vi "Write Library Data.vi"(4 "Library Path":path, 6 "Icon data":T1={"Text Visible?"=FALSE, "Text Opacity"=0, "Templ Visible?"=FALSE, "Templ Opacity"=0, "Relative Path from 1 to 2"=path "", "Image"=bytes[0], "All User Layers"=[], "Body Text"={"Line 1 text"="", "Line 2 text"="", "Line 3 text"="", "Line 4 text"="", "Line 1 color"=0, "Line 2 color"=0, "Line 3 color"=0, "Line 4 color"=0, "Body Text Spec"={"Font"="", "Alignment"=0, "Size"=3}, "Center text vertically"=FALSE, "Capitalize Text"=FALSE}} {"Body Text"."Body Text Spec"."Alignment" items=["left", "center", "right"]}, 8 "error in":errorcluster, 11 "Library Icon Data in":refnum<class "Library Icon Data.lvclass">) -> (0 "error out":errorcluster, 3 "Library Icon Data out":refnum<class "Library Icon Data.lvclass">)   [LabVIEW 2020, in "Library Icon Data.lvclass"]
uses:
  Library Icon Data.lvclass
  Library Icon Data.lvclass/Library Icon Data.ctl
  resource/plugins/lv_icon.lvlib
  vi.lib/LabVIEW Icon API/lv_icon/Controls/Font.ctl
  vi.lib/LabVIEW Icon API/lv_icon/Controls/Alignment.ctl
  vi.lib/LabVIEW Icon API/lv_icon/Controls/BodyText.ctl
  vi.lib/LabVIEW Icon API/lv_icon/Classes/Layer/Layer.lvclass
  vi.lib/LabVIEW Icon API/lv_icon/Controls/LabVIEW Icon Stored Information.ctl
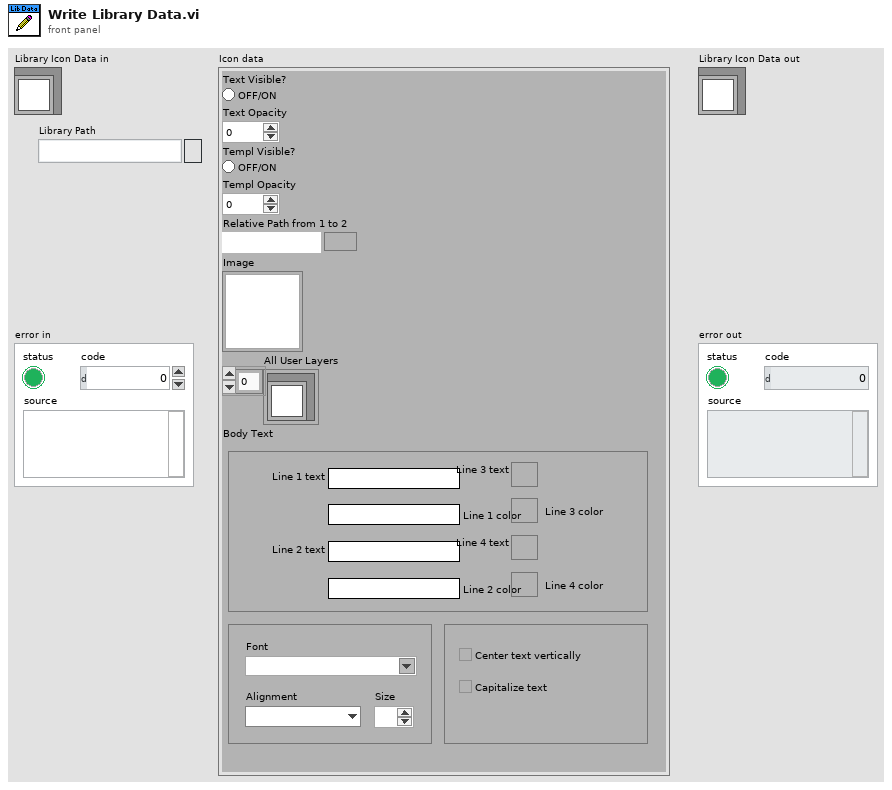
[diagram p1: front panel]
types:
  T1 = typedef "LabVIEW Icon Stored Information.ctl" = cluster{"Text Visible?":bool, "Text Opacity":u8, "Templ Visible?":bool, "Templ Opacity":u8, "Relative Path from 1 to 2":path, "Image":picture, "All User Layers":refnum<class "Layer.lvclass">[], "Body Text":T2}
  T2 = typedef "BodyText.ctl" = cluster{"Line 1 text":string, "Line 2 text":string, "Line 3 text":string, "Line 4 text":string, "Line 1 color":u32, "Line 2 color":u32, "Line 3 color":u32, "Line 4 color":u32, "Body Text Spec":cluster{"Font":T3, "Alignment":T4, "Size":u8}, "Center text vertically":bool, "Capitalize Text":bool}
  T3 = typedef "Font.ctl" = string
  T4 = typedef "Alignment.ctl" = u16
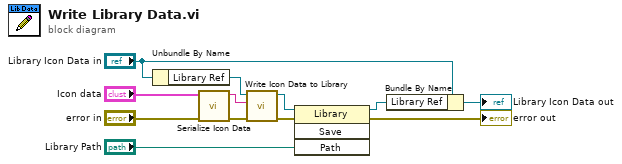
[diagram p0: block diagram]
diagram:
  n1 = Unbundle By Name("Library Icon Data in") -> ("Library Ref"=w7:refnum<vi>)
  n2 = call "Serialize Icon Data.vi"("error in"="error in", "Icon data"="Icon data") -> ("error out"=w12:errorcluster, "data string"=w8:string)  [unwired: 8 in]
  n3 = call "Write Icon Data to Library.vi"("error in"=w12, "Data"=w8, "Library Ref in"=w7) -> ("error out"=w10:errorcluster, "Library Ref out"=w5:refnum<vi>)  [unwired: 7 in]
  n4 = invoke class="Library" method="Save"(reference=w5, error in=w10, "Path"="Library Path") -> (reference out=w3:refnum<vi>, error out=→"error out":errorcluster)  [unwired: 1 in, 2 out]
  n5 = Bundle By Name(cluster="Library Icon Data in", "Library Ref"=w3) -> (→"Library Icon Data out":refnum<class "Library Icon Data.lvclass">)
